vi "DSF.Engine.Memory.Cache.Framework.Get Hardware Specs.vi"(8 "error in (no error)":errorcluster, 11 "Framework Cache in":refnum<class "DSF.Engine.Memory.Cache.Framework.lvclass">) -> (0 "error out":errorcluster, 2 "Hardware Info":T1 {"CPU"."caches"."cache entry size" format="%d bytes"; "CPU"."caches"."total cache size" format="%d bytes"}, 3 "Framework Cache out":refnum<class "DSF.Engine.Memory.Cache.Framework.lvclass">)   [LabVIEW 2016, in "DSF.Engine.lvlib" / "DSF.Engine.Memory.Cache.Framework.lvclass"]
uses:
  DSF.Engine.Memory.Cache.Framework.lvclass
  Framework/DSF.Engine.Runtime.Framework.Hardware.ctl
  Framework/DSF.Engine.Typedefs.CPU Info.ctl
  DSF.Engine.Memory.Cache.Framework.lvclass/DSF.Engine.Memory.Cache.Framework.ctl
  DSF.Engine.lvlib
  Framework/DSF.Engine.Runtime.Framework.lvclass
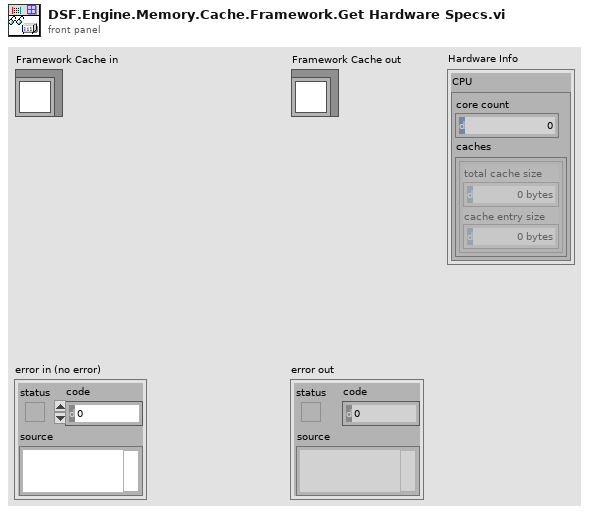
[diagram p1: front panel]
types:
  T1 = typedef "DSF.Engine.lvlib/DSF.Engine.Runtime.Framework.lvclass/DSF.Engine.Runtime.Framework.Hardware.ctl" = cluster{"CPU":T2}
  T2 = typedef "DSF.Engine.lvlib/DSF.Engine.Typedefs.CPU Info.ctl" = cluster{"core count":i32, "caches":cluster{"total cache size":i32, "cache entry size":i32}[]}
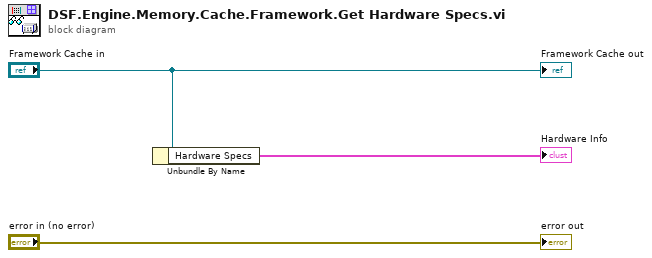
[diagram p0: block diagram]
diagram:
  n1 = Unbundle By Name("Framework Cache in") -> ("Hardware Specs"=→"Hardware Info":T1)
  "error out" <- "error in (no error)"
  "Framework Cache out" <- "Framework Cache in"
